vi "dfd_Wordlength to Text Width.vi"(11 "wl":i16) -> (3 "width":i16)   [LabVIEW 2017, in "NI_DigFilter_Process.lvlib"]
uses:
  <vilib>/addons/Digital Filter Design/NI_DigFilter_Process.lvlib
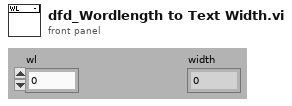
[diagram p1: front panel]
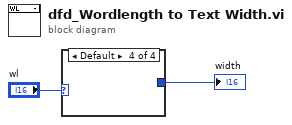
[diagram p0: block diagram]
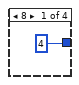
[diagram p2: hidden frame]
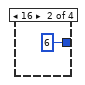
[diagram p3: hidden frame]
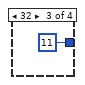
[diagram p4: hidden frame]
diagram:
  n1 = case shown="Default" "wl" {
    tunnel: [4 6 11 _] -> w2
    frame 8 {
    }
    frame 16 {
    }
    frame 32 {
    }
    frame Default {
    }
  }
  "width" <- w2
